vi "Analysis.vi"(8 "error in (no error)":errorcluster, 10 "AllDataToAnal":T1, 11 "PropertiesToOrderAnalysis":T6={"Start/End"=enum."Start", "data"=[], "OrderAnalysis"={"dB on"=FALSE, "window type"=0, "max order to analyze"=0.0, "order resolution"=0.0, "Axis"=0, "Sample rate"=5000, "Save?"=FALSE, "Multiple_Frequency"=3, "averaging mode"=enum."No averaging"}, "Tacho"=[]} {"OrderAnalysis"."Axis" items=["X", "Y", "Z"]; "OrderAnalysis"."window type" items=["No averaging", "Vector averaging", "RMS averaging", "Peak hold"]}) -> (0 "error out":errorcluster, 3 "DataToUI":T4 {"Results"."Mesh_std" format="%#_13g"; "Results"."Mesh_mean" format="%#_13g"; "Results"."Order power spectra"."order 0" format="%.2p"; "Results"."Order power spectra"."delta order" format="%.2p"; "Results"."Order power spectra"."magnitude" format="%.2f"; "Results"."Power Spectrum / PSD"."magnitude" format="%.2p"; "Results"."Power Spectrum / PSD"."f0" format="%.2p"; "Results"."Power Spectrum / PSD"."df" format="%.2p"})   [LabVIEW 2021]
uses:
  <vilib>/measure/NI_MAPro.lvlib
  Typedefs/Results.ctl
  Typedefs/DataToUI.ctl
  Typedefs/Detected peaks.ctl
  <vilib>/measure/matone.llb/Extract Single Tone Information 1 Chan.vi
  <vilib>/addons/Sound and Vibration/Order Analysis/Tach Process/OAT Analog Tacho Process (1 Tacho).vi
  <vilib>/measure/maspectr.llb/FFT Power Spectrum and PSD for N Chan.vi
  <vilib>/addons/Sound and Vibration/Order Analysis/Resample Order Tracking/OAT Convert to Even Angle Signal (N Channels).vi
  <vilib>/addons/Sound and Vibration/Order Analysis/Utility/OAT Output Triggered Even Angle Signal (N Channels).vi
  <vilib>/addons/Sound and Vibration/Order Analysis/Resample Order Tracking/OAT Order Power Spectrum (N Channels).vi
  Typedefs/OrderAnalysis.ctl
  Typedefs/PropertiesOrderAnalysis.ctl
  Typedefs/Start_End.ctl
  Typedefs/Axis.ctl
  Typedefs/PlanetInfo.ctl
  Typedefs/AllDataToAnal.ctl
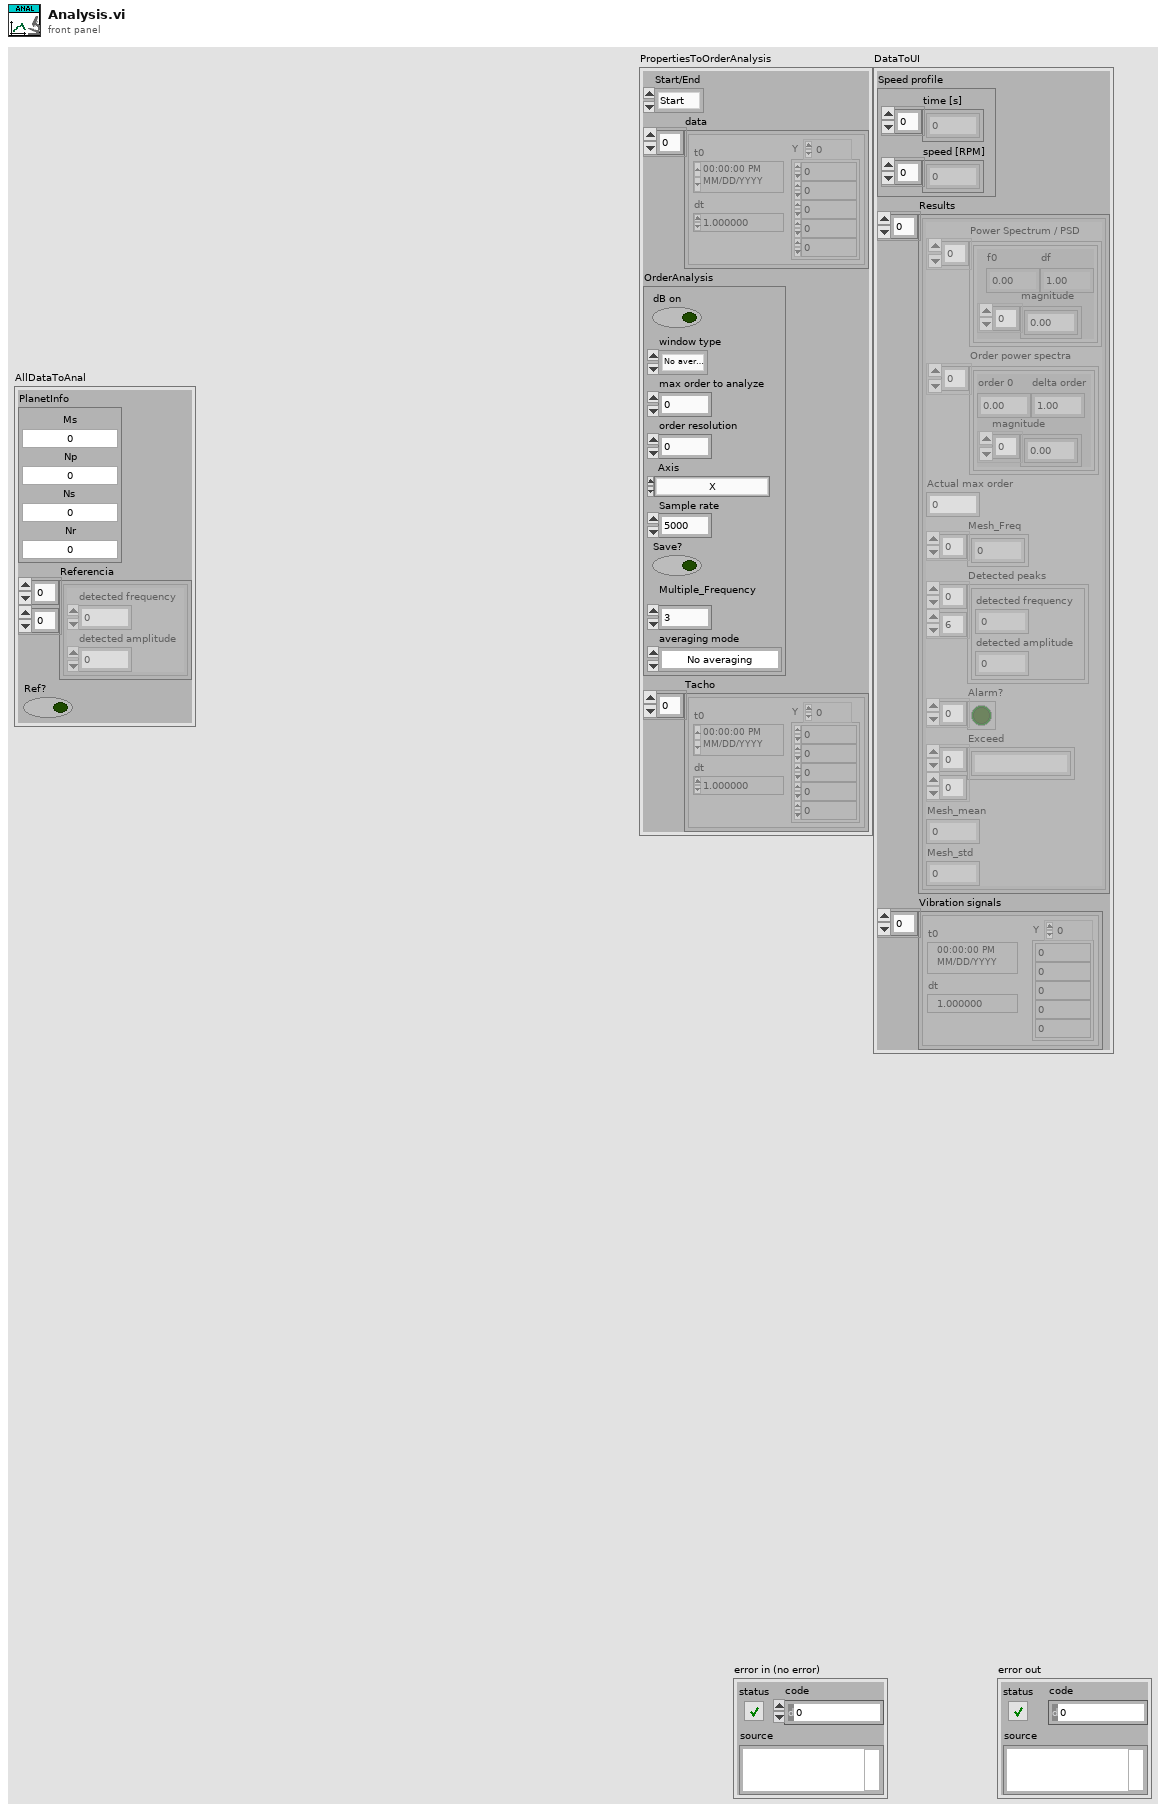
[diagram p1: front panel]
types:
  T1 = typedef "AllDataToAnal.ctl" = cluster{"PlanetInfo":T2, "Referencia":T3[][], "Ref?":bool}
  T2 = typedef "PlanetInfo.ctl" = cluster{"Ms":dbl, "Np":dbl, "Ns":dbl, "Nr":dbl}
  T3 = typedef "Detected peaks.ctl" = cluster{"detected frequency":dbl, "detected amplitude":dbl}
  T4 = typedef "DataToUI.ctl" = cluster{"Speed profile":cluster{"time [s]":dbl[], "speed [RPM]":dbl[]}, "Results":T5[], "Vibration signals":waveform(dbl)[]}
  T5 = typedef "Results.ctl" = cluster{"Power Spectrum / PSD":cluster{"f0":dbl, "df":dbl, "magnitude":dbl[]}[], "Order power spectra":cluster{"order 0":dbl, "delta order":dbl, "magnitude":dbl[]}[], "Actual max order":dbl, "Mesh_Freq":dbl[], "Detected peaks":T3[][], "Alarm?":bool[], "Exceed":string[][], "Mesh_mean":dbl, "Mesh_std":dbl}
  T6 = typedef "PropertiesOrderAnalysis.ctl" = cluster{"Start/End":T7, "data":waveform(dbl)[], "OrderAnalysis":T8, "Tacho":waveform(dbl)[]}
  T7 = typedef "Start_End.ctl" = enum16{"Start", "End"}
  T8 = typedef "OrderAnalysis.ctl" = cluster{"dB on":bool, "window type":u32, "max order to analyze":dbl, "order resolution":dbl, "Axis":T9, "Sample rate":i64, "Save?":bool, "Multiple_Frequency":i32, "averaging mode":enum16{"No averaging", "Vector averaging", "RMS averaging", "Peak hold"}}
  T9 = typedef "Axis.ctl" = u16
  T10 = cluster{"averaging mode":enum16{"No averaging", "Vector averaging", "RMS averaging", "Peak hold"}, "weighting mode":enum16{"Linear", "Exponential"}, "number of averages":u32, "linear mode":enum16{"One shot", "Auto restart"}}
  T11 = enum16{"No averaging", "Vector averaging", "RMS averaging", "Peak hold"}
  T12 = typedef "SoundVib_TachProcess.lvlib/speed profile.ctl" = cluster{"time [s]":dbl[], "speed [RPM]":dbl[]}
  T13 = typedef "svc_Resampled Channel Info.ctl" = cluster{"channel name":string, "description":string, " channel info":T14}
  T14 = typedef "svc_Channel Info.ctl" = cluster{"sensor sensitivity":dbl, "engineering units":T15, "dB reference":dbl, "custom label":string, "weighting filter":T16, "pregain":dbl}
  T15 = typedef "svc_Engineering Units Text Ring.ctl" = u16
  T16 = typedef "svc_Weighting Filter Text Ring.ctl" = u16
  T17 = cluster{"order 0":dbl, "delta order":dbl, "magnitude":dbl[]}[]
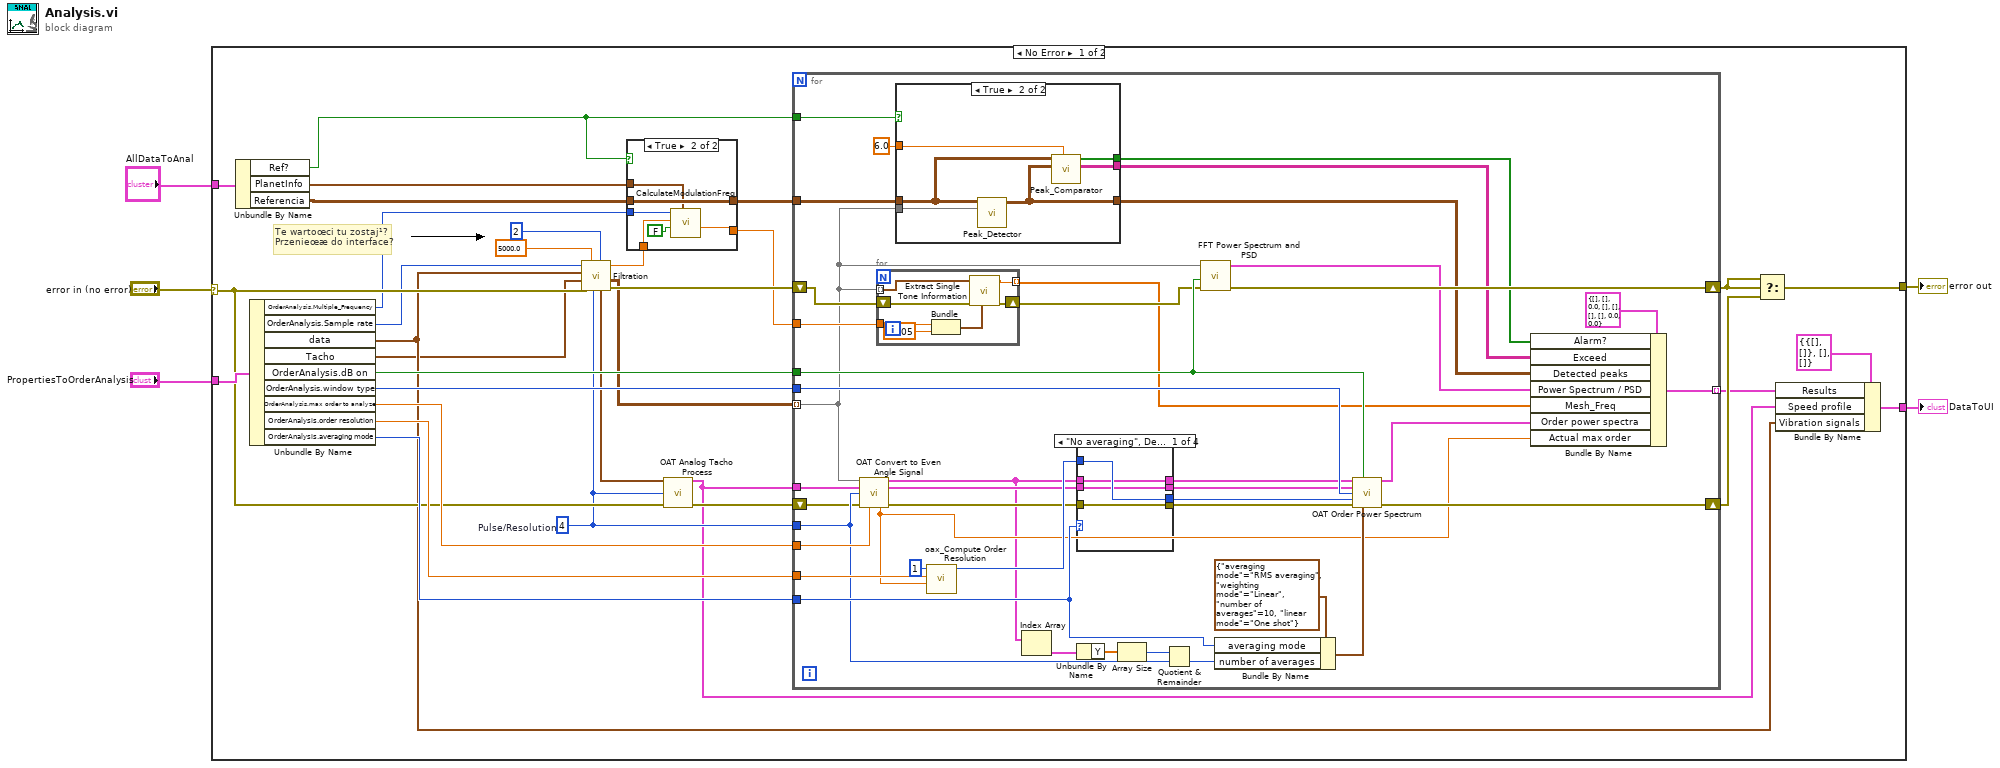
[diagram p0: block diagram]
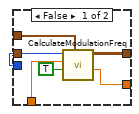
[diagram p2: hidden frame]
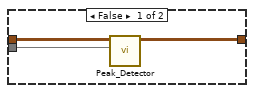
[diagram p3: hidden frame]
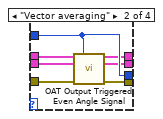
[diagram p4: hidden frame]
diagram:
  n1 = case shown="No Error" "error in (no error)" {
    selector: "error in (no error)" -> [w27 w126]
    tunnel: "PropertiesToOrderAnalysis" -> [w32 _]
    tunnel: [w31 w126] -> w4
    tunnel: [w17 _] -> w2
    tunnel: "AllDataToAnal" -> [w12 _]
    frame No Error {
      w24 = 4  # Pulse/Resolution
      # "Te wartoœci tu zostaj¹?\nPrzenieœæ do interface?"
      n2 = Unbundle By Name(w12) -> ("Ref?"=w10:bool, "PlanetInfo"=w9:T2, "Referencia"=w11:T3[][])
      n3 = Unbundle By Name(w32) -> ("OrderAnalysis.Multiple_Frequency"=w13:i32, "OrderAnalysis.Sample rate"=w26:i64, "data"=w8:waveform(dbl)[], "Tacho"=w7:waveform(dbl)[], "OrderAnalysis.dB on"=w37:bool, "OrderAnalysis.window type"=w33:u32, "OrderAnalysis.max order to analyze"=w34:dbl, "OrderAnalysis.order resolution"=w35:dbl, "OrderAnalysis.averaging mode"=w36:T11)
      n4 = call "Filtration.vi"("order"=2, "Pulse/Resolution"=w24, "low cutoff freq [Hz]"=5000.0, "error in (no error)"=w27, "Tacho in"=w7, "Data in"=w8, "Sample rate"=w26) -> ("error out"=w23:errorcluster, "Data out"=w21:waveform(dbl)[][], "speed [rpm]"=w15:dbl, "Tacho out"=w6:waveform(dbl))  [unwired: 1 in]
      n5 = case shown="True" w10 {
        tunnel: [w43 w49] -> w16
        tunnel: w11 -> [_ w49]
        tunnel: w15 -> [w42 w47]
        tunnel: [w41 w46] -> w14
        tunnel: w13 -> [w39 w45]
        tunnel: w9 -> [w38 w44]
        frame False {
          n6 = call "CalculateModulationFreq.vi"("PlanetInfo"=w38, "All freq"=TRUE, "speed [rpm]"=w42, "Multiple_Frequency"=w39) -> ("Mesh_Freq"=w41:dbl, "char freqs out"=w43:T3[][])  [unwired: 5 in, 1 out]
        }
        frame True {
          n7 = call "CalculateModulationFreq.vi"("PlanetInfo"=w44, "All freq"=FALSE, "speed [rpm]"=w47, "Multiple_Frequency"=w45) -> ("Mesh_Freq"=w46:dbl)  [unwired: 5 in, 2 out]
        }
      }
      n8 = call-poly <vilib>:"OAT Analog Tacho Process.vi"("analog tacho signal"=w6, "pulse/revolution (1)"=w24, "error in (no error)"=w27) -> ("speed profile"=w18:T12, "error out"=w29:errorcluster)  [unwired: 8 in, 3 out]
      n9 = for {
        tunnel: w37 -> [w90]
        tunnel: w36 -> [w89]
        tunnel: w35 -> [w88]
        tunnel: w34 -> [w87]
        tunnel: w33 -> [w86]
        tunnel: w24 -> [w81]
        tunnel: w18 -> [w79]
        shift-right: [w84] -> w30
        shift-left: w23 -> [w55]
        shift-right: [w85] -> w22
        shift-left: w29 -> [w78]
        tunnel: w21 -> [w50] mode=indexing
        tunnel: [w63] -> w19 mode=indexing
        tunnel: w16 -> [w62]
        tunnel: w10 -> [w61]
        tunnel: w14 -> [w53]
        n10 = call-poly <vilib>:"OAT Convert to Even Angle Signal.vi"("scaled signals [EU]"=w50, "speed profile"=w79, "pulse/revolution (1)"=w81, "error in (no error)"=w78, "max order (auto)"=w87) -> ("even-angle signals"=w51:cluster{"r0":dbl, "dr":dbl, "Y":dbl[]}[], "even-angle channel info"=w74:T13[], "actual max order"=w64:dbl, "error out"=w77:errorcluster)  [unwired: 6 in, 1 out]
        n11 = for {
          tunnel: w53 -> [w94]
          shift-right: [w95] -> w54
          shift-left: w55 -> [w96]
          tunnel: w50 -> [w92] mode=indexing
          tunnel: [w91] -> w52 mode=indexing
          n12 = Bundle("Mesh_Freq"=w94, 0.005) -> (w93:cluster{"Mesh_Freq":dbl, dbl})  [unwired: 1 in]
          n13 = call-poly <vilib>:"Extract Single Tone Information.vi"("advanced search"=w93, "error in (no error)"=w96, "time signal in"=w92) -> ("error out"=w95:errorcluster, "detected frequency"=w91:dbl)  [unwired: 3 in, 4 out]
        }
        n14 = case shown="True" w61 {
          tunnel: w50 -> [w100 w106]
          tunnel: w62 -> [w99 w105]
          tunnel: 6.0 ("threshold") -> [_ w102]
          tunnel: [w98 w103] -> w59
          tunnel: [_ w104] -> w56
          tunnel: [_ w101] -> w57
          frame False {
            n15 = call "Peak_Detector.vi"("Data in"=w100, "Referencia"=w99) -> ("Detected peaks"=w98:T3[][])  [unwired: 9 in]
          }
          frame True {
            n16 = call "Peak_Detector.vi"("Data in"=w106, "Referencia"=w105) -> ("Detected peaks"=w103:T3[][])  [unwired: 9 in]
            n17 = call "Peak_Comparator.vi"("threshold"=w102, "Detected peaks"=w103, "Reference peaks"=w105) -> ("Przekroczenia"=w101:string[][], "Alarm?"=w104:bool[])  [unwired: 7 in]
          }
        }
        n18 = call <vilib>:"oax_Compute Order Resolution.vi"("actual max order"=w64, "order resolution"=w88, "block size"=1) -> ("block size out"=w83:i32)  [unwired: 7 in, 1 out]
        n19 = Index Array(array=w51) -> (element=w71:cluster{"r0":dbl, "dr":dbl, "Y":dbl[]})  [unwired: 1 in]
        n20 = case shown="\"No averaging\", Default" w89 {
          tunnel: w77 -> [w109 w117 w118 w122]
          tunnel: [w109 w116 w118 w122] -> w76
          tunnel: w83 -> [w110 w115 w119 w125]
          tunnel: [w110 w115 w119 w125] -> w75
          tunnel: w51 -> [w107 w114 w121 w124]
          tunnel: w74 -> [w108 w113 w120 w123]
          tunnel: [w108 w111 w120 w123] -> w73
          tunnel: [w107 w112 w121 w124] -> w72
          frame "No averaging", Default {
          }
          frame "Vector averaging" {
            n21 = call-poly <vilib>:"OAT Output Triggered Even Angle Signal.vi"("even-angle signals"=w114, "block size"=w115, "even-angle channel info"=w113, "error in (no error)"=w117) -> ("triggered even-angle signals"=w112:cluster{"r0":dbl, "dr":dbl, "Y":dbl[]}[], "even-angle channel info out"=w111:T13[], "error out"=w116:errorcluster)  [unwired: 9 in]
          }
          frame "RMS averaging" {
          }
          frame "Peak hold" {
          }
        }
        n22 = Unbundle By Name(w71) -> ("Y"=w70:dbl[])
        n23 = Array Size(array=w70) -> (size(s)=w69:i32)
        n24 = Quotient & Remainder(x=w69, y=w81) -> (floor(x/y)=w68:i32)  [unwired: 1 out]
        n25 = call-poly <vilib>:"FFT Power Spectrum and PSD.vi"("error in (no error)"=w54, "dB On (F)"=w90, "time signals"=w50) -> ("error out"=w84:errorcluster, "Power Spectrum / PSD"=w66:cluster{"f0":dbl, "df":dbl, "magnitude":dbl[]}[])  [unwired: 5 in, 2 out]
        n26 = Bundle By Name(cluster=T10 {"averaging mode"=enum."RMS averaging", "weighting mode"=enum."Linear", "number of averages"=10, "linear mode"=enum."One shot"} ("averaging parameters"), "averaging mode"=w89, "number of averages"=w68) -> (w67:T10)
        n27 = call-poly <vilib>:"OAT Order Power Spectrum.vi"("even-angle signals"=w72, "dB on? (T)"=w90, "even-angle channel info"=w73, "window"=w86, "block size"=w75, "error in (no error)"=w76, "averaging parameters"=w67) -> ("order power spectra"=w65:T17, "error out"=w85:errorcluster)  [unwired: 2 in, 5 out]
        n28 = Bundle By Name(cluster=T5 {"Power Spectrum / PSD"=[], "Order power spectra"=[], "Actual max order"=0.0, "Mesh_Freq"=[], "Detected peaks"=[], "Alarm?"=[], "Exceed"=[], "Mesh_mean"=0.0, "Mesh_std"=0.0} ("input cluster"), "Alarm?"=w56, "Exceed"=w57, "Detected peaks"=w59, "Power Spectrum / PSD"=w66, "Mesh_Freq"=w52, "Order power spectra"=w65, "Actual max order"=w64) -> (w63:T5)
      }
      n29 = Select(t=w30, s=w30, f=w22) -> (s? t:f=w31:errorcluster)
      n30 = Bundle By Name(cluster=T4 {"Speed profile"={"time [s]"=[], "speed [RPM]"=[]}, "Results"=[], "Vibration signals"=[]}, "Results"=w19, "Speed profile"=w18, "Vibration signals"=w8) -> (w17:T4)
    }
    frame Error {
    }
  }
  "error out" <- w4
  "DataToUI" <- w2
